vi "Timing.Create.vi"(8 "error in (no error)":errorcluster, 9 "Offset":u64, 10 "Decimation":u64=1, 11 "Priority":u64) -> (0 "error out":errorcluster, 3 "Timing":refnum<class "Timing.lvclass">)   [LabVIEW 2017, in "DSF.Engine.lvlib" / "Timing.lvclass"]
uses:
  Timing.lvclass
  Timing.lvclass/Timing.ctl
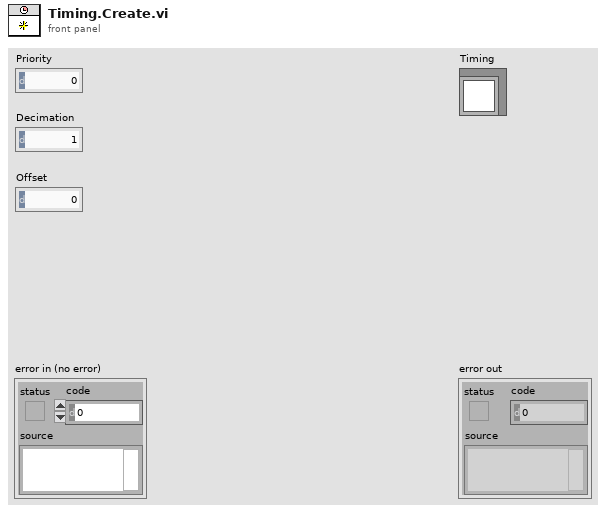
[diagram p1: front panel]
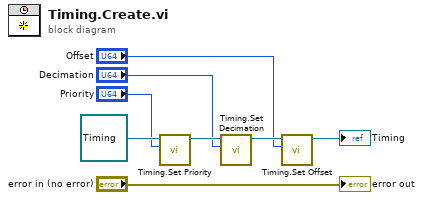
[diagram p0: block diagram]
diagram:
  n1 = call "Timing.Set Priority.vi"("Priority"="Priority", "Timing in"=refnum<class "Timing.lvclass"> refnum ("Timing")) -> ("Timing out"=w6:refnum<class "Timing.lvclass">)  [unwired: 9 in]
  n2 = call "Timing.Set Decimation.vi"("Decimation"="Decimation", "Timing in"=w6) -> ("Timing out"=w4:refnum<class "Timing.lvclass">)  [unwired: 9 in]
  n3 = call "Timing.Set Offset.vi"("Offset"="Offset", "Timing in"=w4) -> ("Timing out"=→"Timing":refnum<class "Timing.lvclass">)  [unwired: 9 in]
  "error out" <- "error in (no error)"
